vi "Analysis.LevelTransition.ODH.vi"(9 "Numeric":dbl, 10 "LVTransitionParameters":T1, 11 "Array in":dbl[][](array[numeric])) -> (3 "Array out":bool[](array[boolean]))   [LabVIEW 2014, in "NIAnalysis.lvlib"]
uses:
  NIAnalysis.lvlib
  Types/Public.LVAnalysis.ctl
  Types/Public.ChLVAnalysis.ctl
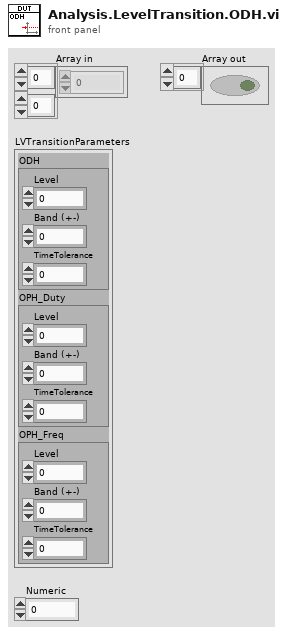
[diagram p1: front panel]
types:
  T1 = typedef "NIAnalysis.lvlib/Public.LVAnalysis.ctl" = cluster{"ODH":T2, "OPH_Duty":T2, "OPH_Freq":T2}
  T2 = typedef "NIAnalysis.lvlib/Public.ChLVAnalysis.ctl" = cluster{"Level":dbl, "Band (+-)":dbl, "TimeTolerance":dbl}
  T3 = cluster{"Scale":dbl, "Hi":dbl, "Lo":dbl, "dt":dbl, "Timeout":dbl}
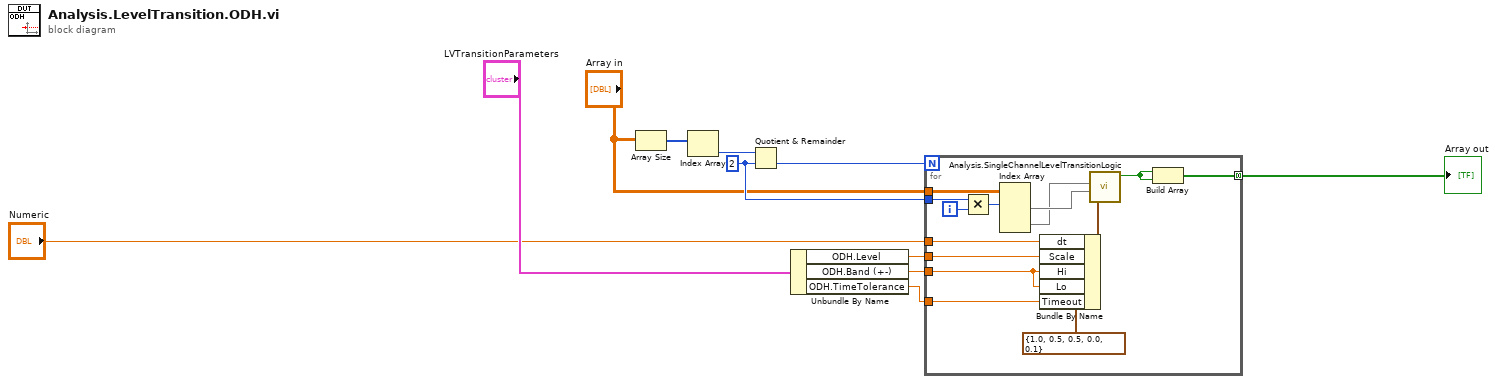
[diagram p0: block diagram]
diagram:
  w5 = 2 ("y")
  n1 = Array Size(array="Array in") -> (size(s)=w2:i32[])
  n2 = Index Array(array=w2) -> (element=w3:i32)  [unwired: 1 in]
  n3 = Quotient & Remainder(x=w3, y=w5) -> (floor(x/y)=w4:i32)  [unwired: 1 out]
  n4 = Unbundle By Name("LVTransitionParameters") -> ("ODH.Level"=w8:dbl, "ODH.Band (+-)"=w9:dbl, "ODH.TimeTolerance"=w10:dbl)
  n5 = for {
    N: w4 -> [_]
    tunnel: "Array in" -> [w25]
    tunnel: w5 -> [w18]
    tunnel: [w16] -> w6 mode=concatenating
    tunnel: "Numeric" -> [w15]
    tunnel: w8 -> [w14]
    tunnel: w9 -> [w13]
    tunnel: w10 -> [w12]
    i -> [w20]
    n6 = Multiply(x=w18, y=w20) -> (x*y=w19:i32)
    n7 = Index Array(array=w25, index (row) #1=w19) -> (element #1=w22:dbl[], element #2=w21:dbl[])  [unwired: 3 in]
    n8 = Bundle By Name(cluster=T3 {"Scale"=1.0, "Hi"=0.5, "Lo"=0.5, "dt"=0.0, "Timeout"=0.1} ("Parameters"), "dt"=w15, "Scale"=w14, "Hi"=w13, "Lo"=w13, "Timeout"=w12) -> (w23:T3)
    n9 = call "Analysis.SingleChannelLevelTransitionLogic.vi"("Stimulus"=w22, "Response"=w21, "Parameters"=w23) -> ("Fail"=w17:bool)  [unwired: 8 in]
    n10 = Build Array(w17, w17) -> (w16:bool[])
  }
  "Array out" <- w6
